vi "niDTS GNSS Dut Initialize.vi"(0 "Session Name ()":string, 2 "GNSS Dut Object Type":refnum<class "niDTS GNSS Dut.lvclass">, 5 "Comm Handle":T3, 7 "Logger":T2, 11 "error in (no error)":errorcluster) -> (4 "GNSS Dut Handle":T1, 15 "error out":errorcluster)   [LabVIEW 2014, in "niDTS GNSS.lvlib"]
uses:
  niDTS GNSS.lvlib
  Framework/Comm/Includes/niDTS Comm INC Handle.ctl
  Framework/Comm/Objects/BASE_class/niDTS Comm.lvclass
  Framework/Logger/Includes/niDTS Logger INC Handle.ctl
  Framework/Logger/Objects/BASE_class/niDTS Logger.lvclass
  Objects/BASE_class/niDTS GNSS Dut.lvclass
  Includes/niDTS GNSS Dut INC Handle.ctl
  Framework/Session/Objects/BASE_class/niDTS Session.lvclass
  Framework/niDTS Framework.lvlib
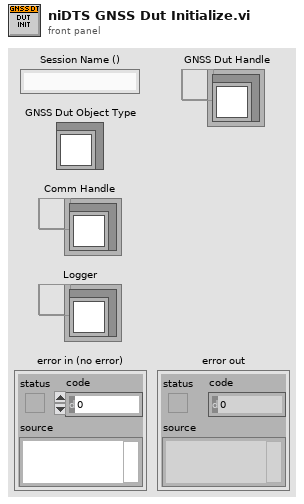
[diagram p1: front panel]
types:
  T1 = typedef "niDTS GNSS.lvlib/niDTS GNSS Dut INC Handle.ctl" = refnum<data-value>
  T2 = typedef "niDTS Framework.lvlib/niDTS Logger INC Handle.ctl" = refnum<data-value>
  T3 = typedef "niDTS Framework.lvlib/niDTS Comm INC Handle.ctl" = refnum<data-value>
  T4 = typedef "niDTS Framework.lvlib/niDTS Session INC Handle.ctl" = refnum<data-value>
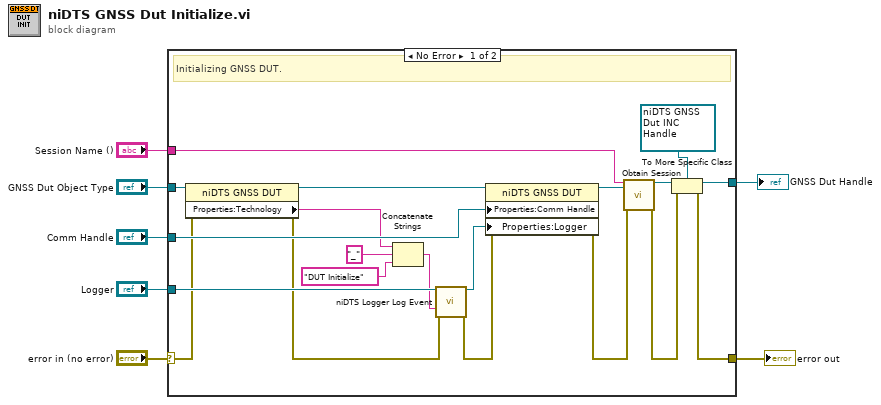
[diagram p0: block diagram]
diagram:
  n1 = case shown="No Error" "error in (no error)" {
    selector: "error in (no error)" -> [w9 w28]
    tunnel: "Session Name ()" -> [w17 _]
    tunnel: [w22 w28] -> w6
    tunnel: [w19 _] -> w1
    tunnel: "Comm Handle" -> [w27 _]
    tunnel: "Logger" -> [w26 _]
    tunnel: "GNSS Dut Object Type" -> [w14 _]
    frame No Error {
      # "Initializing GNSS DUT."
      n2 = property class="niDTS GNSS DUT"(reference=w14, error in=w9) -> (reference out=w15:refnum<class "niDTS GNSS Dut.lvclass">, error out=w8:errorcluster, "Properties:Technology"=w13:string)
      n3 = Concatenate Strings(w13, "_" ("Source/Location"), "DUT Initialize" ("Source/Location")) -> (w12:string)
      n4 = call "niDTS Logger Log Event.vi"("Logger Handle"=w26, "Source/Location"=w12, "error in (no error)"=w8) -> ("Logger Handle out"=w18:T2, "error out"=w23:errorcluster)  [unwired: 10 in, 1 out]
      n5 = property class="niDTS GNSS DUT"(reference=w15, error in=w23, "Properties:Comm Handle"=w27, "Properties:Logger"=w18) -> (reference out=w24:refnum<class "niDTS GNSS Dut.lvclass">, error out=w20:errorcluster)
      n6 = call "Obtain Session.vi"("Session Name ()"=w17, "OBJ - Session"=w24, "error in (no error)"=w20) -> ("Session Handle"=w25:T4, "error out"=w21:errorcluster)  [unwired: 10 in, 1 out]
      n7 = To More Specific Class(target class=T1 refnum ("GPS Dut Handle"), reference=w25, error in=w21) -> (specific class reference=w19:T1, error out=w22:errorcluster)
    }
    frame Error {
    }
  }
  "error out" <- w6
  "GNSS Dut Handle" <- w1
